vi "addForceAndStatusFrame.vi"(8 "error in (no error)":errorcluster, 10 "ModbusBuffer in":refnum<class "ModbusBuffer.lvclass">, 11 "FAILC in":refnum<class "FAILC.lvclass">) -> (0 "error out":errorcluster, 2 "ModbusBuffer out":refnum<class "ModbusBuffer.lvclass">, 3 "FAILC out":refnum<class "FAILC.lvclass">)   [LabVIEW 2016, in "RTFAILC.lvlib" / "FAILC.lvclass"]
uses:
  FAILC.lvclass
  D:/Code/ts_M1M3Support/Common_RT_ILC/ILC/ILC.lvclass
  Common_RT_Modbus/ModbusBuffer/ModbusBuffer.lvclass
  FAILC.lvclass/FAILC.ctl
  Common_RT_ILC/ILC/ILC.lvclass/ILC.ctl
  Common_RT_Modbus/ModbusBuffer/ModbusBuffer.lvclass/ModbusBuffer.ctl
  Common_RT_Modbus/DataTypes/ExceptionCodes.ctl
  Common_RT_Modbus/ModbusBuffer/writeByteInstruction.vi
  Common_RT_Modbus/ModbusBuffer/calculateCRC.vi
  Common_RT_ILC/ILC/ILC.lvclass
  Common_RT_Modbus/RTModbus.lvlib
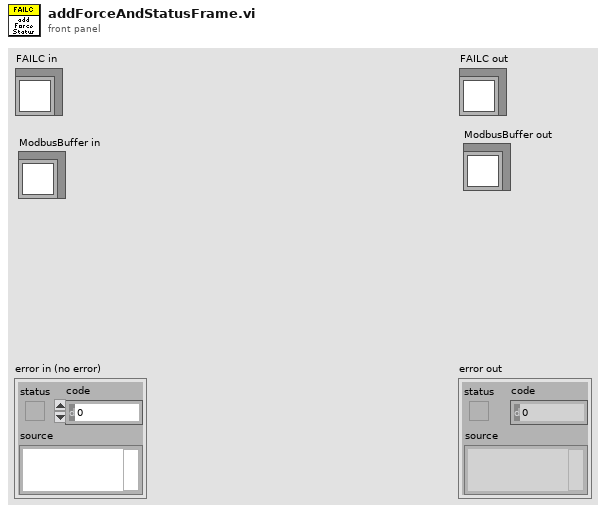
[diagram p1: front panel]
types:
  T1 = typedef "RTModbus.lvlib/ExceptionCodes.ctl" = u16
  T2 = typedef "RTILC.lvlib/ILCData.ctl" = cluster{"Constants":T3, "Command":T4, "Telemetry":T6, "Responses":T7, "Timestamps":T8, "Timings":T9}
  T3 = typedef "RTILC.lvlib/ILCConstants.ctl" = cluster{"Subnet":u8, "Address":u8}
  T4 = typedef "RTILC.lvlib/ILCCommand.ctl" = cluster{"Mode":u16, "TemporaryAddress":u8, "ADCScanRate":T5, "ADCChannel":u8, "ADCOffset":sgl, "ADCSensitivity":sgl}
  T5 = typedef "RTILC.lvlib/ILCScanRates.ctl" = u8
  T6 = typedef "RTILC.lvlib/ILCTelemetry.ctl" = cluster{"UniqueID":u64, "FirmwareType":u8, "NetworkNodeType":u8, "ILCOption":u8, "NetworkNodeOption":u8, "MajorRevision":u8, "MinorRevision":u8, "FirmwareName":string, "Mode":u16, "MajorFault":bool, "MinorFault":bool, "FaultOverride":bool, "MainCalibrationError":bool, "BackupCalibrationError":bool, "UniqueIDCRCMismatch":bool, "AppTypeNodeTypeMismatch":bool, "AppMissing":bool, "AppCRCMismatch":bool, "TEDSNotFound":bool, "TEDS1Mismatch":bool, "TEDS2Mismatch":bool, "WatchdogResetDetected":bool, "BrownoutDetected":bool, "EventTrapResetDetected":bool, "MotorPowerFault":bool, "SSRPowerFault":bool, "AuxPowerFault":bool, "SMCPowerFault":bool, "TemporaryAddress":u8, "ADCScanRate":T5, "MainADCCalibrationK":sgl[], "MainSensorOffset":sgl[], "MainSensorSensitivity":sgl[], "BackupADCCalibrationK":sgl[], "BackupSensorOffset":sgl[], "BackupSensorSensitivity":sgl[]}
  T7 = typedef "RTILC.lvlib/ILCResponses.ctl" = cluster{"ReportServerID":T1, "ReportServerStatus":T1, "Mode":T1, "TemporaryAddress":T1, "Reset":T1, "ADCScanRate":T1, "ADCOffsetSensitivity":T1, "ReportCalibrationData":T1}
  T8 = typedef "RTILC.lvlib/ILCTimestamps.ctl" = cluster{"ReportServerID":dbl, "ReportServerStatus":dbl, "Mode":dbl, "TemporaryAddress":dbl, "Reset":dbl, "ADCScanRate":dbl, "ADCOffsetSensitivity":dbl, "ReportCalibrationData":dbl}
  T9 = typedef "RTILC.lvlib/ILCTimings.ctl" = cluster{"ReportServerID":u32, "ReportServerStatus":u32, "Mode":u32, "TemporaryAddress":u32, "Reset":u32, "ADCScanRate":u32, "ADCOffsetSensitivity":u32, "ReportCalibrationData":u32}
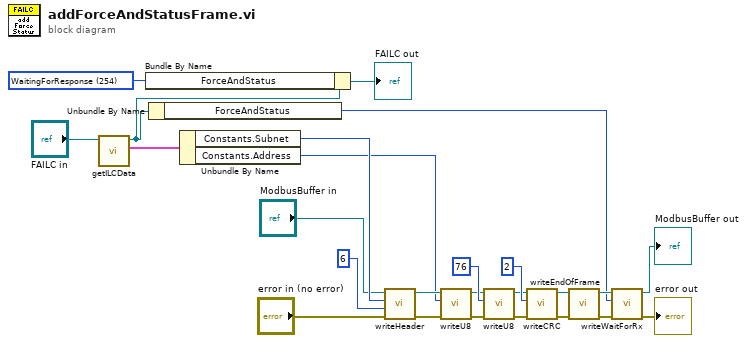
[diagram p0: block diagram]
diagram:
  w6 = T1 254 items=["OK"=0, "IllegalFunction"=1, "IllegalDataAddress"=2, "IllegalDataValue"=3, "SlaveDeviceFailure"=4, "Acknowledge"=5, "SlaveDeviceBusy"=6, "NegativeAcknowledge"=7, "MemoryParityError"=8, "GatewayPathUnavailable"=9, "GatewayTargetDeviceFailedToRespond"=10, "WaitingForResponse"=254, "CRCError"=255] ("FAData.Responses.ForceAndStatus")
  n1 = call "getILCData.vi"("ILC in"="FAILC in") -> ("ILCData"=w25:T2, "ILC out"=w8:refnum<class "FAILC.lvclass">)  [unwired: 9 in]
  n2 = Bundle By Name(cluster=w8, "ForceAndStatus"=w6) -> (→"FAILC out":refnum<class "FAILC.lvclass">)
  n3 = Unbundle By Name(w8) -> ("ForceAndStatus"=w9:u32)
  n4 = Unbundle By Name(w25) -> ("Constants.Subnet"=w16:u8, "Constants.Address"=w15:u8)
  n5 = call "writeHeader.vi"("error in (no error)"="error in (no error)", "Length"=u16 6, "Subnet"=w16, "ModbusBuffer in"="ModbusBuffer in") -> ("error out"=w19:errorcluster, "ModbusBuffer out"=w22:refnum<class "ModbusBuffer.lvclass">)  [unwired: 6 in]
  n6 = call "writeU8.vi"("error in (no error)"=w19, "Input"=w15, "ModbusBuffer in"=w22) -> ("error out"=w18:errorcluster, "ModbusBuffer out"=w14:refnum<class "ModbusBuffer.lvclass">)  [unwired: 7 in]
  n7 = call "writeU8.vi"("error in (no error)"=w18, "Input"=u8 76 ("Function"), "ModbusBuffer in"=w14) -> ("error out"=w1:errorcluster, "ModbusBuffer out"=w4:refnum<class "ModbusBuffer.lvclass">)  [unwired: 7 in]
  n8 = call "writeCRC.vi"("error in (no error)"=w1, "Length"=2, "ModbusBuffer in"=w4) -> ("error out"=w2:errorcluster, "ModbusBuffer out"=w3:refnum<class "ModbusBuffer.lvclass">)  [unwired: 7 in]
  n9 = call "writeEndOfFrame.vi"("error in (no error)"=w2, "ModbusBuffer in"=w3) -> ("error out"=w17:errorcluster, "ModbusBuffer out"=w21:refnum<class "ModbusBuffer.lvclass">)  [unwired: 8 in]
  n10 = call "writeWaitForRx.vi"("error in (no error)"=w17, "Timeout(us)"=w9, "ModbusBuffer in"=w21) -> ("error out"=→"error out":errorcluster, "ModbusBuffer out"=→"ModbusBuffer out":refnum<class "ModbusBuffer.lvclass">)  [unwired: 7 in]
